vi "Line Intersection.vi"(10 "Line 2":T1 {"Point 2"."Y" format="%.2f"; "Point 2"."X" format="%.2f"; "Point 1"."Y" format="%.2f"; "Point 1"."X" format="%.2f"}, 11 "Line 1":T1 {"Point 2"."Y" format="%.2f"; "Point 2"."X" format="%.2f"; "Point 1"."Y" format="%.2f"; "Point 1"."X" format="%.2f"}) -> (3 "Intersection Point":cluster{"X":sgl, "Y":sgl} {"Y" format="%.2f"; "X" format="%.2f"})   [LabVIEW 2025]
uses:
  <vilib>/Analysis/baseanly.llb/Real Determinant.vi
  <vilib>/Analysis/NI_AALBase.lvlib
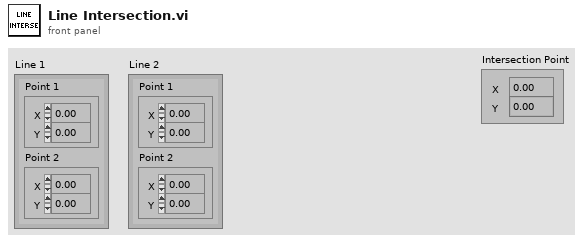
[diagram p1: front panel]
types:
  T1 = cluster{"Point 1":cluster{"X":sgl, "Y":sgl}, "Point 2":cluster{"X":sgl, "Y":sgl}}
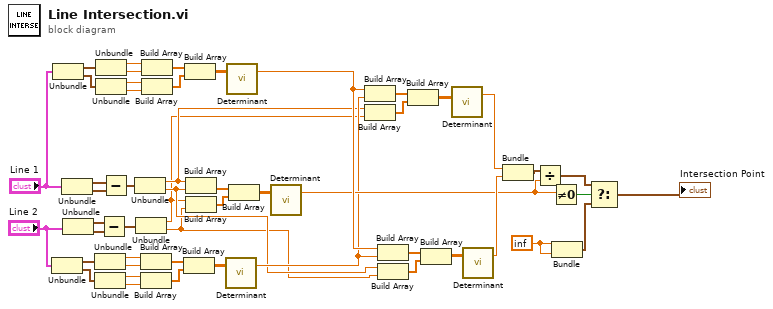
[diagram p0: block diagram]
diagram:
  w24 = inf
  n1 = Unbundle("Line 2") -> ("Point 1"=w32:cluster{"X":sgl, "Y":sgl}, "Point 2"=w33:cluster{"X":sgl, "Y":sgl})
  n2 = Unbundle("Line 1") -> ("Point 1"=w45:cluster{"X":sgl, "Y":sgl}, "Point 2"=w44:cluster{"X":sgl, "Y":sgl})
  n3 = Unbundle("Line 1") -> ("Point 1"=w50:cluster{"X":sgl, "Y":sgl}, "Point 2"=w47:cluster{"X":sgl, "Y":sgl})
  n4 = Unbundle("Line 2") -> ("Point 1"=w48:cluster{"X":sgl, "Y":sgl}, "Point 2"=w49:cluster{"X":sgl, "Y":sgl})
  n5 = Unbundle(w32) -> ("X"=w34:sgl, "Y"=w6:sgl)
  n6 = Unbundle(w33) -> ("X"=w7:sgl, "Y"=w35:sgl)
  n7 = Unbundle(w45) -> ("X"=w43:sgl, "Y"=w8:sgl)
  n8 = Unbundle(w44) -> ("X"=w9:sgl, "Y"=w42:sgl)
  n9 = Subtract(x=w48, y=w49) -> (x-y=w29:cluster{"X":sgl, "Y":sgl})
  n10 = Subtract(x=w50, y=w47) -> (x-y=w30:cluster{"X":sgl, "Y":sgl})
  n11 = Unbundle(w30) -> ("X"=w2:sgl, "Y"=w4:sgl)
  n12 = Unbundle(w29) -> ("X"=w1:sgl, "Y"=w3:sgl)
  n13 = Build Array(w34, w6) -> (w36:sgl[])
  n14 = Build Array(w7, w35) -> (w37:sgl[])
  n15 = Build Array(w43, w8) -> (w41:sgl[])
  n16 = Build Array(w9, w42) -> (w40:sgl[])
  n17 = Build Array(w36, w37) -> (w38:sgl[][])
  n18 = Build Array(w41, w40) -> (w39:sgl[][])
  n19 = Build Array(w2, w4) -> (w27:sgl[])
  n20 = Build Array(w1, w3) -> (w26:sgl[])
  n21 = call-poly <vilib>:"Determinant.vi"("Input Matrix"=w38) -> ("determinant"=w5:dbl)  [unwired: 1 in, 1 out]
  n22 = call-poly <vilib>:"Determinant.vi"("Input Matrix"=w39) -> ("determinant"=w17:dbl)  [unwired: 1 in, 1 out]
  n23 = Build Array(w27, w26) -> (w28:sgl[][])
  n24 = call-poly <vilib>:"Determinant.vi"("Input Matrix"=w28) -> ("determinant"=w11:dbl)  [unwired: 1 in, 1 out]
  n25 = Build Array(w17, w5) -> (w21:dbl[])
  n26 = Build Array(w2, w1) -> (w22:sgl[])
  n27 = Build Array(w17, w5) -> (w19:dbl[])
  n28 = Build Array(w4, w3) -> (w18:sgl[])
  n29 = Build Array(w21, w22) -> (w20:dbl[][])
  n30 = Build Array(w19, w18) -> (w16:dbl[][])
  n31 = call-poly <vilib>:"Determinant.vi"("Input Matrix"=w20) -> ("determinant"=w15:dbl)  [unwired: 1 in, 1 out]
  n32 = call-poly <vilib>:"Determinant.vi"("Input Matrix"=w16) -> ("determinant"=w14:dbl)  [unwired: 1 in, 1 out]
  n33 = Bundle("determinant"=w15, "determinant"=w14) -> (w12:cluster{"determinant":dbl, "determinant":dbl})  [unwired: 1 in]
  n34 = Divide(x=w12, y=w11) -> (x/y=w10:cluster{"determinant":dbl, "determinant":dbl})
  n35 = Not Equal To 0?(x=w11) -> (x != 0?=w25:bool)
  n36 = Bundle(w24, w24) -> (w13:cluster{dbl, dbl})  [unwired: 1 in]
  n37 = Select(t=w10, s=w25, f=w13) -> (s? t:f=→"Intersection Point":cluster{"determinant":dbl, "determinant":dbl})
